vi "CopyFromDVR.vi"(8 "error in":errorcluster, 11 "node in":refnum<data-value>) -> (0 "error out":errorcluster, 2 "CEF_Node out":refnum<class "CEF_Node.lvclass">, 3 "node out":refnum<data-value>)   [LabVIEW 2023, in "CEF.lvlib" / "CEF_Node.lvclass"]
doc: "Copyright 2017 National Instruments Corporation\n\nLicensed under the Apache License, Version 2.0 (the \"License\"); you may not use this file except in compliance with the License. You may obtain a copy of the License at http://www.apache.org/licenses/LICENSE-2.0\nUnless required by applicable law or agreed to in writing, software distributed under the License is distributed on an \"AS IS\" BASIS, WITHOUT WARRANTIES OR CONDITIONS OF ANY KIND, either express or implied. See the License for the specific language governing permissions and limitations under the License."
uses:
  CEF_Node.lvclass
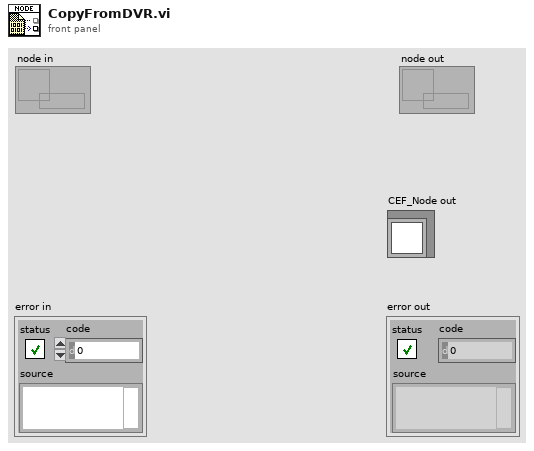
[diagram p1: front panel]
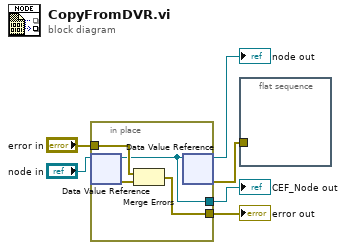
[diagram p0: block diagram]
diagram:
  n1 = in-place {
    in-place-border: "error in" -> [w10]
    in-place-border: [w9] -> w5
    in-place-border: [w7] -> w1
    n2 = in-place-dvr #1("node in") -> (w7:refnum<class "CEF_Node.lvclass">, w8:errorcluster)
    n3 = Merge Errors(w10, w8) -> (w9:errorcluster)
    n4 = in-place-dvr #1(w7) -> (→"node out":refnum<data-value>, w2:errorcluster)
  }
  "error out" <- w5
  "CEF_Node out" <- w1
  n5 = flat-sequence {
    tunnel: w2 -> [_]
    frame #0 {
    }
  }
